vi "main.vi"() -> ()   [LabVIEW 2015, in "example_02.lvlib"]
uses:
  example_02.lvlib
  _controls/customer.ctl
  _controls/tab_control.ctl
  <userlib>/antonio-alexander/lv-recipe-machine/public/_controls/mode.ctl
  <userlib>/antonio-alexander/lv-recipe-machine/public/_controls/automatic_state.ctl
  <userlib>/antonio-alexander/lv-recipe-machine/public/_controls/configuration.ctl
  _controls/fg_command.ctl
  <userlib>/antonio-alexander/lv-recipe-machine/lv-recipe-machine.lvlib
panel:
  out "step_elapsed_time":dbl format="%<%H:%M:%S>t"
  out "recipe_elapsed_time":dbl format="%<%H:%M:%S>t"
  out "step":string
  out "automatic_data":variant
  out "automatic_state":T1
  out "mode":T2
  in  "begin":bool
  out "error":errorcluster
  in  "exit":bool
  in  "next":bool
  in  "previous":bool
  in  "submit":bool
  out "tab_control":T3=enum."begin"
  in  "first_name":string
  in  "last_name":string
  in  "address_1":string
  in  "address_2":string
  in  "city":string
  in  "state":string
  in  "zip_code":string
  out "customer":T4
  # "Click submit to finish"
  # "Click submit to finish"
  # "Click begin to start"
  # "Click begin to start"
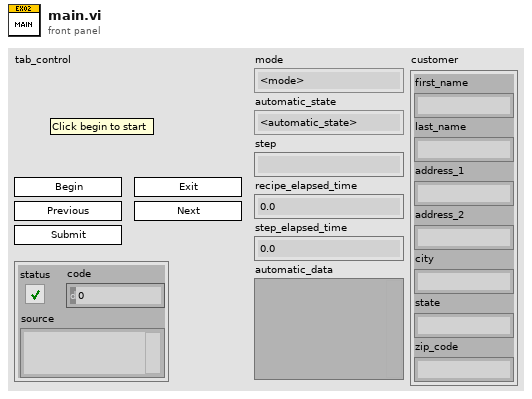
[diagram p1: front panel]
types:
  T1 = typedef "lv-recipe-machine.lvlib/automatic_state.ctl" = enum16{"<automatic_state>", "failed", "idle", "running", "paused", "stopped", "<null>"}
  T2 = typedef "lv-recipe-machine.lvlib/mode.ctl" = enum16{"<mode>", "manual", "automatic", "<null>"}
  T3 = typedef "example_02.lvlib/tab_control.ctl" = enum32{"first_name", "last_name", "address", "city", "state", "zip_code", "submit", "begin"}
  T4 = typedef "example_02.lvlib/customer.ctl" = cluster{"first_name":string, "last_name":string, "address_1":string, "address_2":string, "city":string, "state":string, "zip_code":string}
  T5 = typedef "example_02.lvlib/fg_command.ctl" = enum16{"<fg_command>", "initialize", "read", "write", "shutdown"}
  T6 = typedef "lv-recipe-machine.lvlib/configuration.ctl" = cluster{"change_in_timeout_ms":i32}
  T7 = cluster{"change_out":refnum<event-registration>, "status_event_registration":refnum<event-registration>}
  T8 = typedef "lv-recipe-machine.lvlib/recipe_step.ctl" = cluster{"step":string, "data":variant}
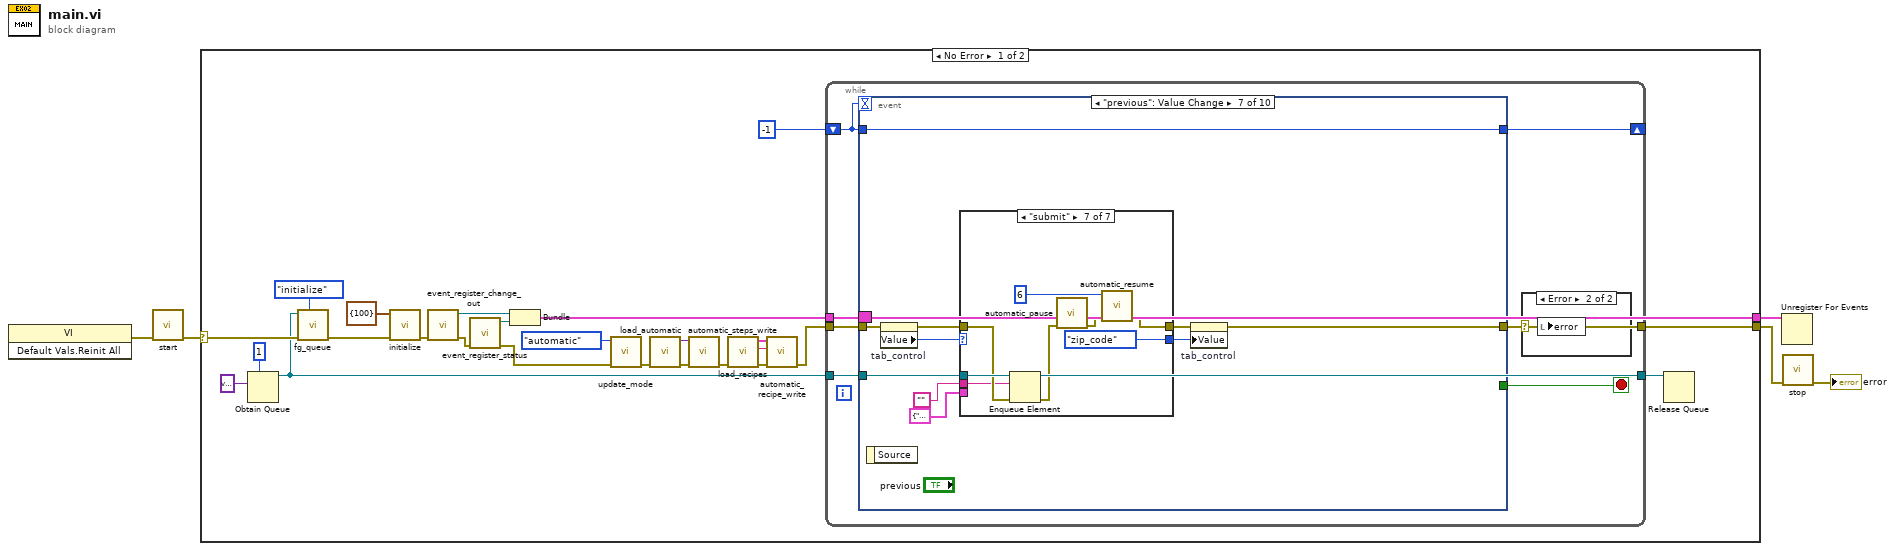
[diagram p0: block diagram]
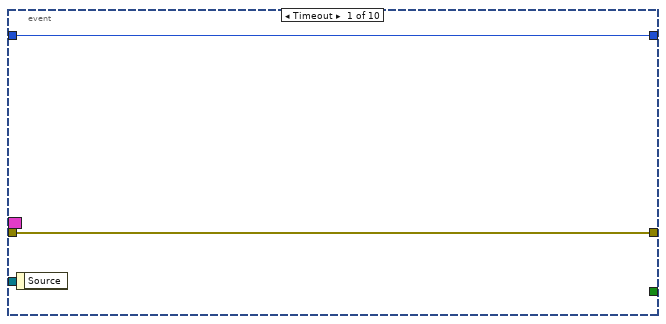
[diagram p3: hidden frame]
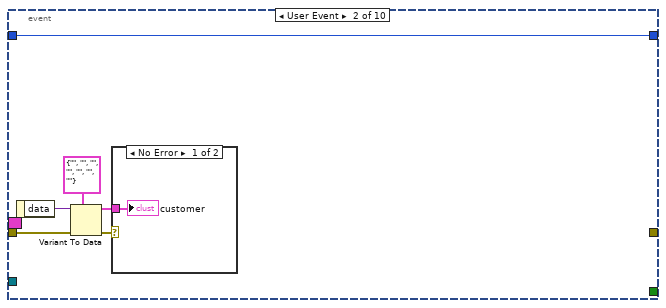
[diagram p4: hidden frame]
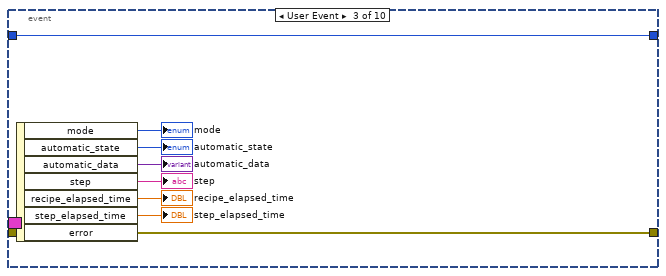
[diagram p6: hidden frame]
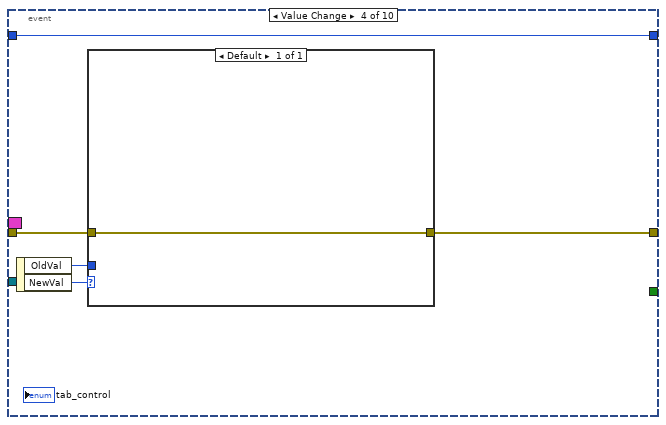
[diagram p7: hidden frame]
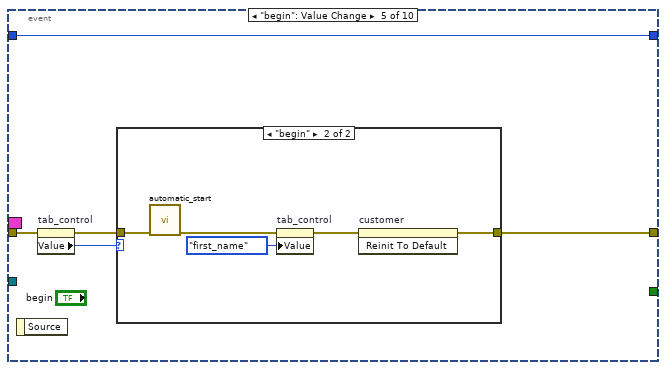
[diagram p8: hidden frame]
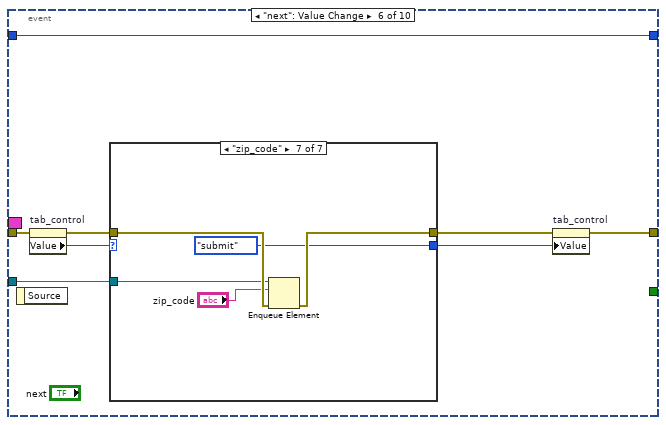
[diagram p10: hidden frame]
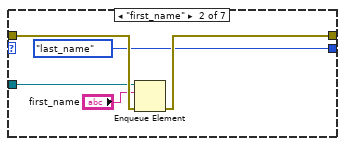
[diagram p12: hidden frame]
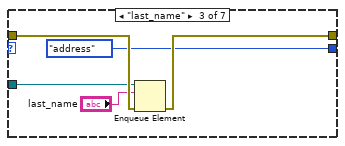
[diagram p13: hidden frame]
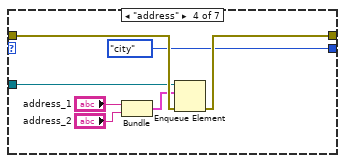
[diagram p14: hidden frame]
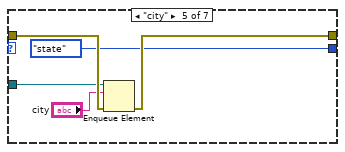
[diagram p15: hidden frame]
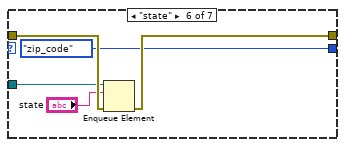
[diagram p16: hidden frame]
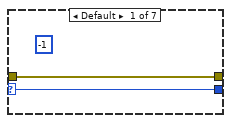
[diagram p17: hidden frame]
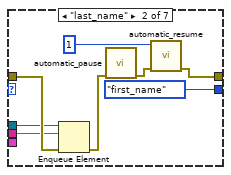
[diagram p18: hidden frame]
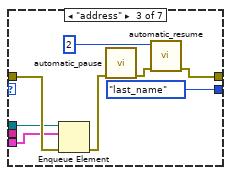
[diagram p19: hidden frame]
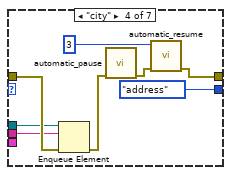
[diagram p20: hidden frame]
diagram:
  n1 = invoke class="VI" method="Default Vals.Reinit All"() -> (error out=w5:errorcluster)  [unwired: 3 in, 2 out]
  n2 = call <userlib>:"start.vi"("error in (no error)"=w5) -> ("error out"=w2:errorcluster)  [unwired: 10 in]
  n3 = case shown="No Error" w2 {
    selector: w2 -> [w30 w194]
    tunnel: [w23 w194] -> w4
    tunnel: [w22 _] -> w1
    frame No Error {
      n4 = Obtain Queue(max queue size (-1, unlimited)=1, element data type=variant) -> (queue out=w6:refnum<queue>)  [unwired: 3 in, 2 out]
      n5 = call "fg_queue.vi"("command"=fg_command."initialize", "error in (no error)"=w30, "queue in"=w6) -> ("error out"=w11:errorcluster)  [unwired: 7 in, 1 out]
      n6 = call <userlib>:"initialize.vi"("error in (no error)"=w11, "configuration"=T6 {"change_in_timeout_ms"=100}) -> ("error out"=w14:errorcluster)  [unwired: 9 in]
      n7 = call <userlib>:"event_register_change_out.vi"("error in (no error)"=w14) -> ("error out"=w24:errorcluster, "change_out"=w26:refnum<event-registration>)  [unwired: 9 in]
      n8 = call <userlib>:"event_register_status.vi"("error in (no error)"=w24) -> ("error out"=w13:errorcluster, "status_event_registration"=w25:refnum<event-registration>)  [unwired: 9 in]
      n9 = Bundle("change_out"=w26, "status_event_registration"=w25) -> (w22:T7)  [unwired: 1 in]
      n10 = call <userlib>:"update_mode.vi"("error in (no error)"=w13, "mode"=mode."automatic") -> ("error out"=w16:errorcluster)  [unwired: 9 in]
      n11 = call "load_automatic.vi"("error in (no error)"=w16) -> ("error out"=w28:errorcluster, "automatic_steps out"=w27:variant)  [unwired: 8 in, 1 out]
      n12 = call <userlib>:"automatic_steps_write.vi"("error in (no error)"=w28, "automatic_steps"=w27) -> ("error out"=w17:errorcluster)  [unwired: 8 in, 1 out]
      n13 = call "load_recipes.vi"("error in (no error)"=w17) -> ("error out"=w18:errorcluster, "transition []"=w19:string, "recipe []"=w20:T8[])  [unwired: 8 in]
      n14 = call <userlib>:"automatic_recipe_write.vi"("error in (no error)"=w18, "transition"=w19, "recipe []"=w20) -> ("error out"=w12:errorcluster)  [unwired: 8 in]
      n15 = while {
        tunnel: w12 -> [w36]
        tunnel: [w35] -> w23
        tunnel: w22 -> [w34]
        shift-right: [w33] -> _
        shift-left: -1 -> [w32]
        tunnel: w6 -> [w31]
        tunnel: [w31] -> w8
        stop <- w37 stop-if-true
        n16 = event shown="[6] \"previous\": Value Change" {
          selector: w34 -> [_ _ _ _ _ _ _ _ _ _]
          dyn-events: _ -> [_ _ _ _ _ _ _ _ _ _]
          timeout: w32 -> [_ _ _ _ _ _ _ _ _ _]
          tunnel: [_ _ _ _ _ _ _ _ w190 TRUE] -> w37
          tunnel: w36 -> [w39 w44 _ w57 w64 w79 w123 w180 _ w191]
          tunnel: [w39 _ w48 w56 w65 w76 w122 w179 _ w191] -> w35
          tunnel: w32 -> [w40 w46 w55 w60 w66 w80 w124 w181 w189 w192]
          tunnel: [w40 w46 w55 w60 w66 w80 w124 w181 w189 w192] -> w33
          tunnel: w31 -> [_ _ _ _ _ w74 w118 w176 _ _]
          event Timeout {
            n17 = event-data() -> ()  [unwired: 1 in, 1 out]
          }
          event User Event {
            n18 = event-data() -> ("data"=w45:variant)  [unwired: 1 in]
            n19 = Variant To Data(error in=w44, type=T4 {"first_name"="", "last_name"="", "address_1"="", "address_2"="", "city"="", "state"="", "zip_code"=""} ("customer"), Variant=w45) -> (data=w43:T4, error out=w41:errorcluster)
            n20 = case shown="No Error" w41 {
              tunnel: w43 -> [w47 _]
              frame No Error {
                "customer" <- w47
              }
              frame Error {
              }
            }
          }
          event User Event {
            n21 = event-data() -> ("mode"=→"mode":T2, "automatic_state"=→"automatic_state":T1, "automatic_data"=→"automatic_data":variant, "step"=→"step":string, "recipe_elapsed_time"=→"recipe_elapsed_time":dbl, "step_elapsed_time"=→"step_elapsed_time":dbl, "error"=w48:errorcluster)  [unwired: 1 in]
          }
          event Value Change {
            n22 = event-data() -> ("OldVal"=w58:T3, "NewVal"=w59:T3)  [unwired: 1 in]
            n23 = case shown="Default" w59 {
              tunnel: w58 -> [_]
              tunnel: w57 -> [w61]
              tunnel: [w61] -> w56
              frame Default {
              }
            }
          }
          event "begin": Value Change {
            n24 = event-data() -> ()  [unwired: 1 in, 1 out]
            n25 = property on="tab_control" class="TabCtl (strict)"(error in=w64) -> (error out=w63:errorcluster, "Value"=w62:T3)  [unwired: 1 in, 1 out]
            n26 = case shown="\"begin\"" w62 {
              tunnel: [w67 w68] -> w65
              tunnel: w63 -> [w67 w70]
              frame Default {
              }
              frame "begin" {
                n27 = call <userlib>:"automatic_start.vi"("error in (no error)"=w70) -> ("error out"=w72:errorcluster)  [unwired: 10 in]
                n28 = property on="tab_control" class="TabCtl (strict)"(error in=w72, "Value"=tab_control."first_name" ("tab_control")) -> (error out=w69:errorcluster)  [unwired: 1 in, 1 out]
                n29 = invoke on="customer" class="Clust (strict)" method="Reinit To Default"(error in=w69) -> (error out=w68:errorcluster)  [unwired: 2 in, 2 out]
              }
            }
          }
          event "next": Value Change {
            n30 = event-data() -> ()  [unwired: 1 in, 1 out]
            n31 = property on="tab_control" class="TabCtl (strict)"(error in=w79) -> (error out=w77:errorcluster, "Value"=w78:T3)  [unwired: 1 in, 1 out]
            n32 = case shown="\"zip_code\"" w78 {
              selector: w78 -> [w81 _ _ _ _ _ _]
              tunnel: w77 -> [w82 w87 w92 w99 w104 w109 w114]
              tunnel: [w82 w86 w91 w98 w103 w108 w113] -> w73
              tunnel: [w81 tab_control."last_name" ("tab_control") tab_control."address" ("tab_control") tab_control."city" ("tab_control") tab_control."state" ("tab_control") tab_control."zip_code" ("tab_control") tab_control."submit" ("tab_control")] -> w75
              tunnel: w74 -> [_ w84 w89 w96 w101 w106 w111]
              frame Default {
              }
              frame "first_name" {
                n33 = Enqueue Element(queue=w84, element="first_name", error in (no error)=w87) -> (error out=w86:errorcluster)  [unwired: 1 in, 2 out]
              }
              frame "last_name" {
                n34 = Enqueue Element(queue=w89, element="last_name", error in (no error)=w92) -> (error out=w91:errorcluster)  [unwired: 1 in, 2 out]
              }
              frame "address" {
                n35 = Bundle("address_1"="address_1", "address_2"="address_2") -> (w95:cluster{"address_1":string, "address_2":string})  [unwired: 1 in]
                n36 = Enqueue Element(queue=w96, element=w95, error in (no error)=w99) -> (error out=w98:errorcluster)  [unwired: 1 in, 2 out]
              }
              frame "city" {
                n37 = Enqueue Element(queue=w101, element="city", error in (no error)=w104) -> (error out=w103:errorcluster)  [unwired: 1 in, 2 out]
              }
              frame "state" {
                n38 = Enqueue Element(queue=w106, element="state", error in (no error)=w109) -> (error out=w108:errorcluster)  [unwired: 1 in, 2 out]
              }
              frame "zip_code" {
                n39 = Enqueue Element(queue=w111, element="zip_code", error in (no error)=w114) -> (error out=w113:errorcluster)  [unwired: 1 in, 2 out]
              }
            }
            n40 = property on="tab_control" class="TabCtl (strict)"(error in=w73, "Value"=w75) -> (error out=w76:errorcluster)  [unwired: 1 in, 1 out]
          }
          event "previous": Value Change {
            n41 = event-data() -> ()  [unwired: 1 in, 1 out]
            n42 = property on="tab_control" class="TabCtl (strict)"(error in=w123) -> (error out=w120:errorcluster, "Value"=w121:T3)  [unwired: 1 in, 1 out]
            n43 = case shown="\"submit\"" w121 {
              selector: w121 -> [w125 _ _ _ _ _ _]
              tunnel: w120 -> [w126 w134 w142 w150 w158 w166 w174]
              tunnel: [w125 tab_control."first_name" ("tab_control") tab_control."last_name" ("tab_control") tab_control."address" ("tab_control") tab_control."city" ("tab_control") tab_control."state" ("tab_control") tab_control."zip_code" ("tab_control")] -> w119
              tunnel: [w126 w127 w136 w144 w152 w160 w168] -> w115
              tunnel: "" -> [_ w132 _ w143 w151 w159 w167]
              tunnel: w118 -> [_ w131 w140 w148 w156 w164 w172]
              tunnel: cluster{string, string} {"", ""} -> [_ _ w135 _ _ _ _]
              frame Default {
                (unwired) -1
              }
              frame "last_name" {
                n44 = Enqueue Element(queue=w131, element=w132, error in (no error)=w134) -> (error out=w128:errorcluster)  [unwired: 1 in, 2 out]
                n45 = call <userlib>:"automatic_pause.vi"("error in (no error)"=w128) -> ("error out"=w129:errorcluster)  [unwired: 10 in]
                n46 = call <userlib>:"automatic_resume.vi"("error in (no error)"=w129, "index"=1) -> ("error out"=w127:errorcluster)  [unwired: 9 in]
              }
              frame "address" {
                n47 = Enqueue Element(queue=w140, element=w135, error in (no error)=w142) -> (error out=w137:errorcluster)  [unwired: 1 in, 2 out]
                n48 = call <userlib>:"automatic_pause.vi"("error in (no error)"=w137) -> ("error out"=w138:errorcluster)  [unwired: 10 in]
                n49 = call <userlib>:"automatic_resume.vi"("error in (no error)"=w138, "index"=2) -> ("error out"=w136:errorcluster)  [unwired: 9 in]
              }
              frame "city" {
                n50 = Enqueue Element(queue=w148, element=w143, error in (no error)=w150) -> (error out=w145:errorcluster)  [unwired: 1 in, 2 out]
                n51 = call <userlib>:"automatic_pause.vi"("error in (no error)"=w145) -> ("error out"=w146:errorcluster)  [unwired: 10 in]
                n52 = call <userlib>:"automatic_resume.vi"("error in (no error)"=w146, "index"=3) -> ("error out"=w144:errorcluster)  [unwired: 9 in]
              }
              frame "state" {
                n53 = Enqueue Element(queue=w156, element=w151, error in (no error)=w158) -> (error out=w153:errorcluster)  [unwired: 1 in, 2 out]
                n54 = call <userlib>:"automatic_pause.vi"("error in (no error)"=w153) -> ("error out"=w154:errorcluster)  [unwired: 10 in]
                n55 = call <userlib>:"automatic_resume.vi"("error in (no error)"=w154, "index"=4) -> ("error out"=w152:errorcluster)  [unwired: 9 in]
              }
              frame "zip_code" {
                n56 = Enqueue Element(queue=w164, element=w159, error in (no error)=w166) -> (error out=w161:errorcluster)  [unwired: 1 in, 2 out]
                n57 = call <userlib>:"automatic_pause.vi"("error in (no error)"=w161) -> ("error out"=w162:errorcluster)  [unwired: 10 in]
                n58 = call <userlib>:"automatic_resume.vi"("error in (no error)"=w162, "index"=5) -> ("error out"=w160:errorcluster)  [unwired: 9 in]
              }
              frame "submit" {
                n59 = Enqueue Element(queue=w172, element=w167, error in (no error)=w174) -> (error out=w169:errorcluster)  [unwired: 1 in, 2 out]
                n60 = call <userlib>:"automatic_pause.vi"("error in (no error)"=w169) -> ("error out"=w170:errorcluster)  [unwired: 10 in]
                n61 = call <userlib>:"automatic_resume.vi"("error in (no error)"=w170, "index"=6) -> ("error out"=w168:errorcluster)  [unwired: 9 in]
              }
            }
            n62 = property on="tab_control" class="TabCtl (strict)"(error in=w115, "Value"=w119) -> (error out=w122:errorcluster)  [unwired: 1 in, 1 out]
          }
          event "submit": Value Change {
            n63 = event-data() -> ()  [unwired: 1 in, 1 out]
            n64 = property on="tab_control" class="TabCtl (strict)"(error in=w180) -> (error out=w178:errorcluster, "Value"=w177:T3)  [unwired: 1 in, 1 out]
            n65 = case shown="\"submit\"" w177 {
              tunnel: [w182 w187] -> w179
              tunnel: w178 -> [w182 w188]
              tunnel: variant -> [_ w185]
              tunnel: w176 -> [_ w183]
              frame Default {
              }
              frame "submit" {
                n66 = Enqueue Element(queue=w183, element=w185, error in (no error)=w188) -> (error out=w184:errorcluster)  [unwired: 1 in, 2 out]
                n67 = property on="tab_control" class="TabCtl (strict)"(error in=w184, "Value"=tab_control."begin" ("tab_control")) -> (error out=w187:errorcluster)  [unwired: 1 in, 1 out]
              }
            }
          }
          event Panel Close? {
            w190 = TRUE
            n68 = event-data() -> ()  [unwired: 1 in, 1 out]
            n69 = event-data("Discard?"=w190) -> ()  [unwired: 1 in, 1 out]
          }
          event "exit": Value Change {
            n70 = event-data() -> ()  [unwired: 1 in, 1 out]
          }
        }
        n71 = case shown="Error" w35 {
          selector: w35 -> [_ w38]
          frame No Error {
          }
          frame Error {
            n72 = local write "error"(w38) -> ()
          }
        }
      }
      n73 = Release Queue(queue=w8) -> ()  [unwired: 2 in, 3 out]
    }
    frame Error {
    }
  }
  n74 = Unregister For Events(event registration refnum=w1) -> ()  [unwired: 1 in, 1 out]
  n75 = call <userlib>:"stop.vi"("error in (no error)"=w4) -> ("error out"=→"error":errorcluster)  [unwired: 10 in]
